vi "Read DBRef.vi"(8 "error in (no error)":errorcluster, 11 "DatabaseBaseClass in":refnum<class "DatabaseBaseClass.lvclass">) -> (0 "error out":errorcluster, 2 "reference":T1, 3 "DatabaseBaseClass out":refnum<class "DatabaseBaseClass.lvclass">)   [LabVIEW 2018, in "Database.lvlib" / "DatabaseBaseClass.lvclass"]
uses:
  DatabaseBaseClass.lvclass
  <vilib>/addons/database/Connection.llb/Conn ObjectReference.ctl
  DatabaseBaseClass.lvclass/DatabaseBaseClass.ctl
  <vilib>/addons/database/NI_Database_API.lvlib
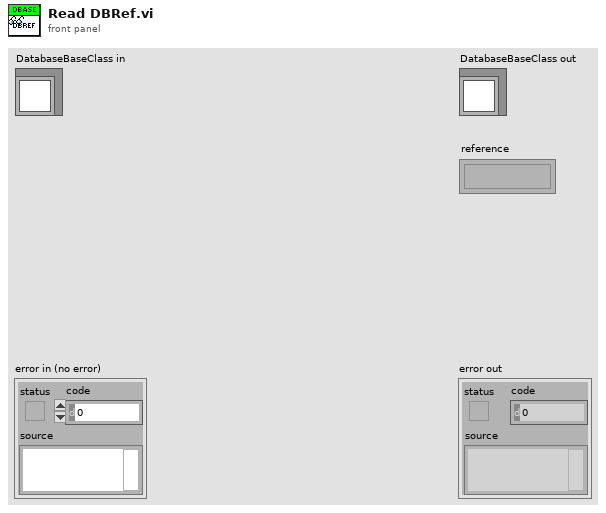
[diagram p1: front panel]
types:
  T1 = typedef "NI_Database_API.lvlib/Conn ObjectReference.ctl" = refnum<k1>
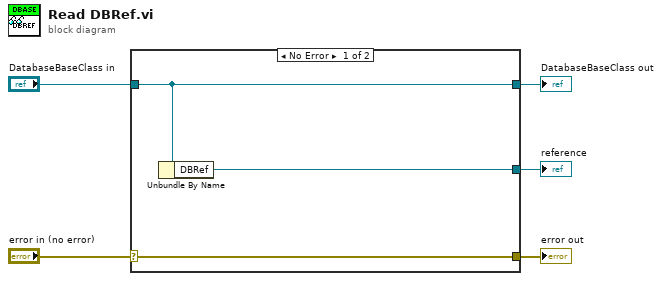
[diagram p0: block diagram]
diagram:
  n1 = case shown="No Error" "error in (no error)" {
    selector: "error in (no error)" -> [w8 w9]
    tunnel: [w8 w9] -> w4
    tunnel: [w7 w10] -> w2
    tunnel: "DatabaseBaseClass in" -> [w7 w10]
    tunnel: [w6 _] -> w1
    frame No Error {
      n2 = Unbundle By Name(w7) -> ("DBRef"=w6:T1)
    }
    frame Error {
    }
  }
  "error out" <- w4
  "DatabaseBaseClass out" <- w2
  "reference" <- w1
